vi "Prueba2_Albi_Cantor_new.vi"() -> ()   [LabVIEW 2013]
panel:
  out "Thermometer":dbl(slide) scale=0.0..220.0
  out "mayor":dbl
  out "Menor":dbl
  out "Temperatura80":dbl
  out "Promedio":dbl
  out "Velocidad":i32(knob) scale=0.0..220.0
  # "Necesitamos generar 10 velocidades. \nal final de las 10 pruebas presentar :\n-Promedio de las velocidades mayores a 120\n-Velocidad Mayor y menor \n-Cuantas veces la temperatura fue mayor a 80"
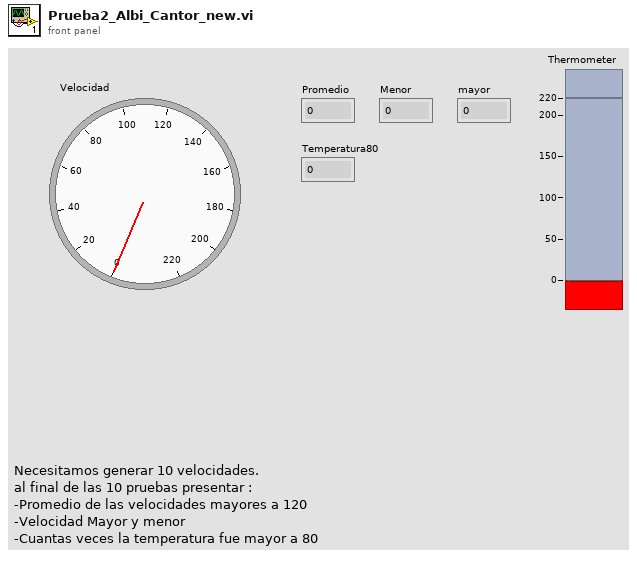
[diagram p1: front panel]
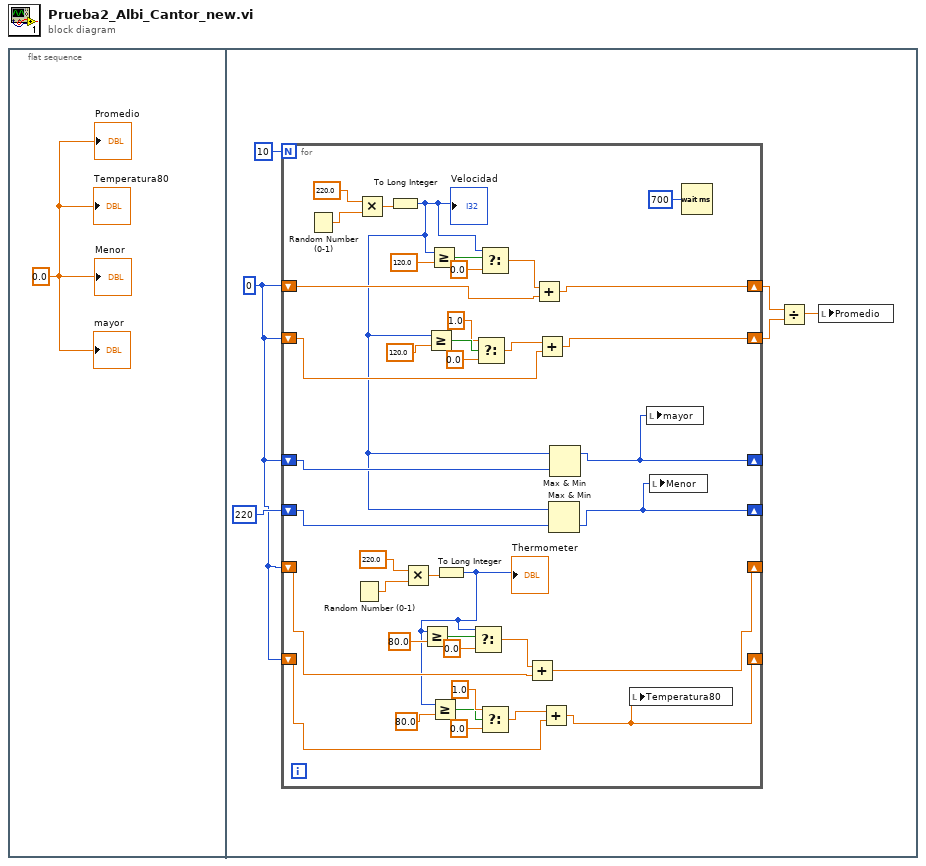
[diagram p0: block diagram]
diagram:
  n1 = flat-sequence {
    frame #0 {
      w1 = 0.0 ("Menor")
      "Promedio" <- w1
      "Temperatura80" <- w1
      "Menor" <- w1
      "mayor" <- w1
    }
    frame #1 {
      w2 = 0
      n2 = for {
        N: 10 -> [_]
        shift-right: [w38] -> w5
        shift-left: w2 -> [w39]
        shift-right: [w31] -> w6
        shift-left: w2 -> [w32]
        shift-right: [w29] -> _
        shift-left: w2 -> [w30]
        shift-right: [w27] -> _
        shift-left: 220 -> [w28]
        shift-right: [w21] -> _
        shift-left: w2 -> [w22]
        shift-right: [w12] -> _
        shift-left: w2 -> [w14]
        n3 = Random Number (0-1)() -> (number: 0 to 1=w45:dbl)
        n4 = Random Number (0-1)() -> (number: 0 to 1=w10:dbl)
        n5 = Multiply(x=220.0, y=w45) -> (x*y=w46:dbl)
        n6 = To Long Integer(number=w46) -> (32bit integer=w15:i32)
        "Velocidad" <- w15
        n7 = Multiply(x=220.0, y=w10) -> (x*y=w9:dbl)
        n8 = Greater Or Equal?(x=w15, y=120.0) -> (x >= y?=w35:bool)
        n9 = Greater Or Equal?(x=w15, y=120.0) -> (x >= y?=w42:bool)
        n10 = To Long Integer(number=w9) -> (32bit integer=w8:i32)
        "Thermometer" <- w8
        n11 = Greater Or Equal?(x=w8, y=80.0) -> (x >= y?=w24:bool)
        n12 = Greater Or Equal?(x=w8, y=80.0) -> (x >= y?=w18:bool)
        n13 = Select(t=w8, s=w24, f=0.0) -> (s? t:f=w26:dbl)
        n14 = Select(t=1.0, s=w35, f=0.0) -> (s? t:f=w33:dbl)
        n15 = Select(t=w15, s=w42, f=0.0) -> (s? t:f=w40:dbl)
        n16 = Select(t=1.0, s=w18, f=0.0) -> (s? t:f=w20:dbl)
        n17 = Add(x=w26, y=w22) -> (x+y=w21:dbl)
        n18 = Add(x=w40, y=w39) -> (x+y=w38:dbl)
        n19 = Add(x=w33, y=w32) -> (x+y=w31:dbl)
        n20 = Add(x=w20, y=w14) -> (x+y=w12:dbl)
        n21 = Max & Min(x=w15, y=w28) -> (min(x,y)=w27:i32)  [unwired: 1 out]
        n22 = Max & Min(x=w15, y=w30) -> (max(x,y)=w29:i32)  [unwired: 1 out]
        n23 = local write "Temperatura80"(w12) -> ()
        n24 = local write "mayor"(w29) -> ()
        n25 = local write "Menor"(w27) -> ()
        n26 = Wait (ms)(milliseconds to wait=u32 700) -> ()  [unwired: 1 out]
      }
      n27 = Divide(x=w5, y=w6) -> (x/y=w4:dbl)
      n28 = local write "Promedio"(w4) -> ()
    }
  }
